vi "CheckIfPeakDetected.vi"(1 "data":waveform(dbl)) -> (0 "Peak detected?":bool)   [LabVIEW 2013]
uses:
  Global.vi
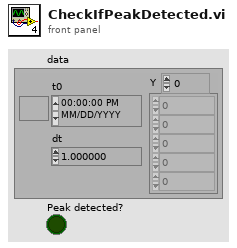
[diagram p1: front panel]
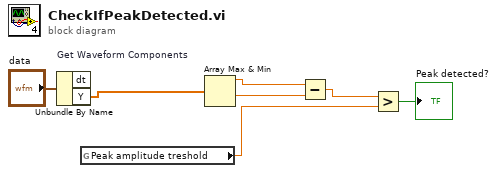
[diagram p0: block diagram]
diagram:
  n1 = Unbundle By Name "Get Waveform Components"("data") -> ("Y"=w6:dbl[])  [unwired: 1 out]
  n2 = global read "Global.vi" "Peak amplitude treshold"() -> (w2:dbl)
  n3 = Array Max & Min(array=w6) -> (max value=w5:dbl, min value=w4:dbl)  [unwired: 2 out]
  n4 = Subtract(x=w5, y=w4) -> (x-y=w3:dbl)
  n5 = Greater?(x=w3, y=w2) -> (0:→"Peak detected?":bool)
